vi "get_files_info.vi"(7 "pattern":string, 8 "error in (no error)":errorcluster, 11 "Folder path in":path) -> (0 "error out":errorcluster, 1 "Number of Files":i32, 2 "All Files in Dir":path[](array[path]), 3 "Folder Path out":path)   [LabVIEW 2015]
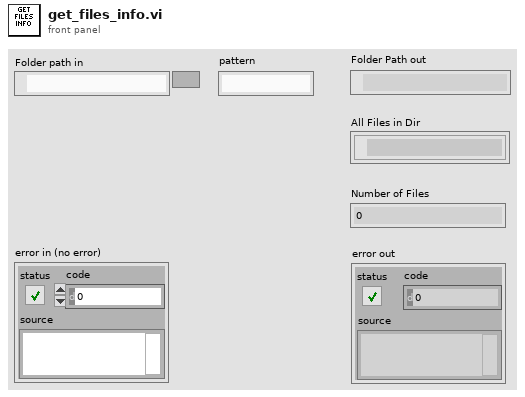
[diagram p1: front panel]
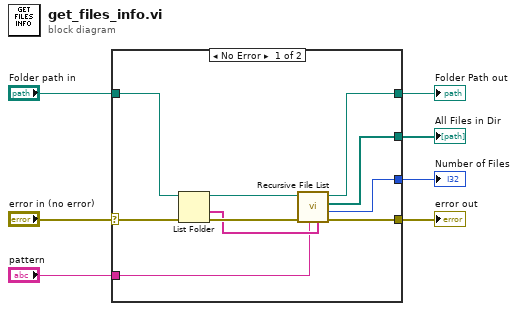
[diagram p0: block diagram]
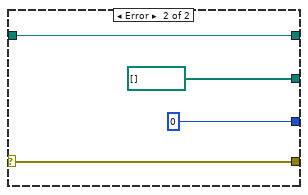
[diagram p2: hidden frame]
diagram:
  n1 = case shown="No Error" "error in (no error)" {
    selector: "error in (no error)" -> [w9 w21]
    tunnel: [w17 0 ("Number of Files")] -> w7
    tunnel: "Folder path in" -> [w13 w20]
    tunnel: [w12 w20] -> w5
    tunnel: [w11 path[] [] ("All Files in Dir")] -> w4
    tunnel: "pattern" -> [w10 _]
    tunnel: [w8 w21] -> w1
    frame No Error {
      n2 = List Folder(path=w13, error in=w9) -> (path out=w15:path, folder names=w14:string[], error out=w16:errorcluster)  [unwired: 2 in, 1 out]
      n3 = call <vilib>:"Recursive File List.vi"("Folders to Exclude"=w14, "pattern"=w10, "error in (no error)"=w16, "Folder Path"=w15) -> ("error out"=w8:errorcluster, "Number of Files"=w17:i32, "All Files in Dir"=w11:path[], "dup Folder Path"=w12:path)  [unwired: 3 in, 1 out]
    }
    frame Error {
    }
  }
  "error out" <- w1
  "Folder Path out" <- w5
  "All Files in Dir" <- w4
  "Number of Files" <- w7
